vi "GE 5565PIORC.DMA.vi"(11 "count (1000)":i32=1000) -> (0 "error out":errorcluster, 3 "pass?":bool)   [LabVIEW 2016]
uses:
  <vilib>/NI/GE Reflective Memory Driver/GE 5565PIORC.lvclass/GE 5565PIORC.ctl
  <vilib>/NI/GE Reflective Memory Driver/Methods/GE 5565PIORC.DMA.Create Transfer (Block).vi
  <vilib>/NI/GE Reflective Memory Driver/Methods/GE 5565PIORC.DMA.Block.Read (DBL).vi
  <vilib>/NI/GE Reflective Memory Driver/Properties/Registers/GE 5565PIORC.Registers.INTCSR.Local DMA Channel 0 Interrupt Enable.Set.vi
  <vilib>/NI/GE Reflective Memory Driver/Properties/Registers/GE 5565PIORC.Registers.INTCSR.PCI Interrupt Enable.Set.vi
  <vilib>/NI/GE Reflective Memory Driver/Properties/Registers/GE 5565PIORC.Registers.INTCSR.Local Interrupt Input Enable.Set.vi
  <vilib>/NI/GE Reflective Memory Driver/Properties/Registers/GE 5565PIORC.Registers.DMACSR0.Channel 0 Enable.Set.vi
  <vilib>/NI/GE Reflective Memory Driver/Methods/GE 5565PIORC.DMA.Create Transfer (Scatter-Gather).vi
  <vilib>/NI/GE Reflective Memory Driver/Methods/GE 5565PIORC.PXI Interrupts.Discard Events.vi
  <vilib>/NI/GE Reflective Memory Driver/Methods/GE 5565PIORC.DMA.Start.vi
  <vilib>/NI/GE Reflective Memory Driver/Methods/GE 5565PIORC.DMA.Wait for Done Interrupt.vi
  <vilib>/NI/GE Reflective Memory Driver/Methods/GE 5565PIORC.VISA.Move In.DBL.vi
  <vilib>/NI/GE Reflective Memory Driver/Properties/Registers/GE 5565PIORC.Registers.Local Configuration.Read.vi
  <vilib>/NI/GE Reflective Memory Driver/Properties/Registers/GE 5565PIORC.Registers.Local Configuration.Read (U32).vi
  <vilib>/NI/GE Reflective Memory Driver/Properties/Registers/GE 5565PIORC.Registers.Local Configuration.Write.vi
  <vilib>/NI/GE Reflective Memory Driver/Properties/Registers/GE 5565PIORC.Registers.Local Configuration.Write (U32).vi
  <vilib>/NI/GE Reflective Memory Driver/Methods/GE 5565PIORC.Bit Manipulation.Set Bit.vi
  <vilib>/NI/GE Reflective Memory Driver/Methods/GE 5565PIORC.Bit Manipulation.Set Bit (U32).vi
  <vilib>/NI/GE Reflective Memory Driver/Properties/Registers/GE 5565PIORC.Registers.Local Configuration.Read (U8).vi
  <vilib>/NI/GE Reflective Memory Driver/Properties/Registers/GE 5565PIORC.Registers.Local Configuration.Write (U8).vi
  <vilib>/NI/GE Reflective Memory Driver/Methods/GE 5565PIORC.Bit Manipulation.Set Bit (U8).vi
  <vilib>/NI/GE Reflective Memory Driver/Methods/GE 5565PIORC.DMA.Size.vi
  <vilib>/Utility/error.llb/Clear Errors.vi
  <vilib>/NI/GE Reflective Memory Driver/Properties/Registers/GE 5565PIORC.Registers.DMACSR0.Channel 0 Start.Set.vi
  <vilib>/NI/GE Reflective Memory Driver/Methods/GE 5565PIORC.PXI Interrupts.Wait for Event.vi
  <vilib>/NI/GE Reflective Memory Driver/Properties/Registers/GE 5565PIORC.Registers.DMACSR0.Channel 0 Clear Interrupt.Set.vi
  <vilib>/NI/GE Reflective Memory Driver/Methods/GE 5565PIORC.VISA.Move In.String (U8).vi
  <vilib>/NI/GE Reflective Memory Driver/Methods/GE 5565PIORC.Registers.Read.vi
  <vilib>/NI/GE Reflective Memory Driver/Methods/GE 5565PIORC.Registers.Read (U32).vi
  <vilib>/NI/GE Reflective Memory Driver/Methods/GE 5565PIORC.Registers.Write.vi
  <vilib>/NI/GE Reflective Memory Driver/Methods/GE 5565PIORC.Registers.Write (U32).vi
  <vilib>/NI/GE Reflective Memory Driver/Methods/GE 5565PIORC.Registers.Read (U8).vi
  <vilib>/NI/GE Reflective Memory Driver/Methods/GE 5565PIORC.Registers.Write (U8).vi
  <vilib>/NI/GE Reflective Memory Driver/Methods/GE 5565PIORC.VISA.Return Handler.vi
  <vilib>/NI/GE Reflective Memory Driver/Methods/GE 5565PIORC.Round Up to Nearest 8.vi
  <vilib>/NI/GE Reflective Memory Driver/Methods/GE 5565PIORC.Round Up to Nearest 16.vi
  <vilib>/NI/GE Reflective Memory Driver/Methods/GE 5565PIORC.DMA.Block.Write (DBL).vi
  <vilib>/NI/GE Reflective Memory Driver/Methods/GE 5565PIORC.DMA.Configure.vi
  <vilib>/Utility/error.llb/Error Cluster From Error Code.vi
  <vilib>/NI/GE Reflective Memory Driver/GE 5565PIORC.lvclass
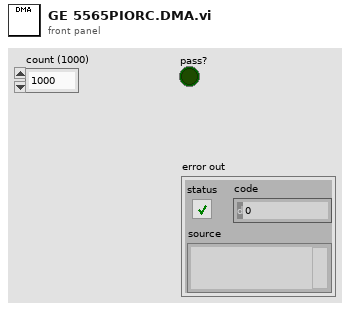
[diagram p1: front panel]
types:
  T1 = typedef "GE 5565PIORC.lvclass/GE 5565PIORC.Typedef.DMA Block Descriptor.ctl" = cluster{"descriptor ptr (VISA)":u32, "descriptor ptr (RFM)":u32, "descriptor size":u32, "descriptor params":T2}
  T2 = typedef "GE 5565PIORC.lvclass/GE 5565PIORC.Typedef.DMA Block Descriptor Params.ctl" = cluster{"data ptr (lower)":u32, "data ptr (upper)":u32, "data size":u32, "next descriptor ptr":u32}
  T3 = typedef "GE 5565PIORC.lvclass/GE 5565PIORC.Typedef.DMA Transfer Spec.ctl" = cluster{"RFM offset":u32, "Block Descriptors":T1[]}
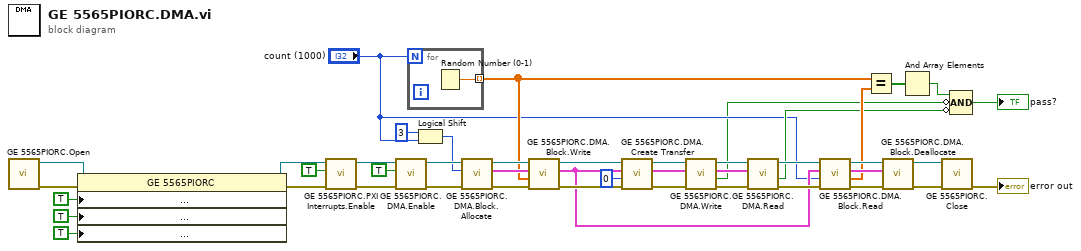
[diagram p0: block diagram]
diagram:
  n1 = call "GE 5565PIORC.Open.vi"() -> ("error out"=w11:errorcluster, "GE 5565PIORC"=w14:refnum<class "GE 5565PIORC.lvclass">)  [unwired: 10 in]
  n2 = property class="GE 5565PIORC"(reference=w14, error in=w11, "Properties:Board Registers:Local Configuration:03 - 0x68 - INTCSR:Local DMA Channel 0 Interrupt Enable"=TRUE ("Registers:Local Configuration:INTCSR:Local DMA Channel 0 Interrupt Enable"), "Properties:Board Registers:Local Configuration:03 - 0x68 - INTCSR:PCI Interrupt Enable"=TRUE ("Registers:Local Configuration:INTCSR:PCI Interrupt Enable"), "Properties:Board Registers:Local Configuration:03 - 0x68 - INTCSR:Local Interrupt Input Enable"=TRUE ("Registers:Local Configuration:INTCSR:Local Interrupt Input Enable")) -> (reference out=w13:refnum<class "GE 5565PIORC.lvclass">, error out=w12:errorcluster)
  n3 = call <vilib>:"GE 5565PIORC.PXI Interrupts.Enable.vi"("error in (no error)"=w12, "Enable Interrupts"=TRUE, "GE 5565PIORC in"=w13) -> ("error out"=w16:errorcluster, "GE 5565PIORC out"=w17:refnum<class "GE 5565PIORC.lvclass">)  [unwired: 7 in]
  n4 = call <vilib>:"GE 5565PIORC.DMA.Enable.vi"("error in (no error)"=w16, "Enable DMA"=TRUE, "GE 5565PIORC in"=w17) -> ("error out"=w41:errorcluster, "GE 5565PIORC out"=w42:refnum<class "GE 5565PIORC.lvclass">)  [unwired: 7 in]
  n5 = for {
    N: "count (1000)" -> [_]
    tunnel: [w45] -> w26 mode=indexing
    n6 = Random Number (0-1)() -> (number: 0 to 1=w45:dbl)
  }
  n7 = Logical Shift(y=i16 3, x="count (1000)") -> (x << y=w36:i32)
  n8 = call <vilib>:"GE 5565PIORC.DMA.Block.Allocate.vi"("error in (no error)"=w41, "size in bytes"=w36, "GE 5565PIORC in"=w42) -> ("error out"=w38:errorcluster, "Block Descriptor"=w37:T1, "GE 5565PIORC out"=w39:refnum<class "GE 5565PIORC.lvclass">)  [unwired: 6 in]
  n9 = call-poly <vilib>:"GE 5565PIORC.DMA.Block.Write.vi"("error in (no error)"=w38, "data"=w26, "Block Descriptor in"=w37, "GE 5565PIORC in"=w39) -> ("error out"=w33:errorcluster, "Block Descriptor out"=w30:T1, "GE 5565PIORC out"=w34:refnum<class "GE 5565PIORC.lvclass">)  [unwired: 4 in, 1 out]
  n10 = call-poly <vilib>:"GE 5565PIORC.DMA.Create Transfer.vi"("error in (no error)"=w33, "RFM offset"=u32 0, "Block Descriptor"=w30, "GE 5565PIORC in"=w34) -> ("error out"=w6:errorcluster, "DMA Transfer Spec"=w5:T3, "GE 5565PIORC out"=w7:refnum<class "GE 5565PIORC.lvclass">)  [unwired: 4 in, 1 out]
  n11 = call <vilib>:"GE 5565PIORC.DMA.Write.vi"("error in (no error)"=w6, "DMA Transfer Spec"=w5, "GE 5565PIORC in"=w7) -> ("error out"=w2:errorcluster, "timed out?"=w1:bool, "DMA Transfer Spec dup"=w4:T3, "GE 5565PIORC out"=w3:refnum<class "GE 5565PIORC.lvclass">)  [unwired: 5 in]
  n12 = call <vilib>:"GE 5565PIORC.DMA.Read.vi"("error in (no error)"=w2, "DMA Transfer Spec"=w4, "GE 5565PIORC in"=w3) -> ("error out"=w31:errorcluster, "timed out?"=w24:bool, "GE 5565PIORC out"=w32:refnum<class "GE 5565PIORC.lvclass">)  [unwired: 5 in, 1 out]
  n13 = call-poly <vilib>:"GE 5565PIORC.DMA.Block.Read.vi"("error in (no error)"=w31, "count"="count (1000)", "Block Descriptor in"=w30, "GE 5565PIORC in"=w32) -> ("error out"=w27:errorcluster, "data out"=w25:dbl[], "Block Descriptor out"=w28:T1, "GE 5565PIORC out"=w29:refnum<class "GE 5565PIORC.lvclass">)  [unwired: 4 in]
  n14 = Equal?(x=w26, y=w25) -> (x = y?=w23:bool[])
  n15 = call <vilib>:"GE 5565PIORC.DMA.Block.Deallocate.vi"("error in (no error)"=w27, "Block Descriptor"=w28, "GE 5565PIORC in"=w29) -> ("error out"=w20:errorcluster, "GE 5565PIORC out"=w21:refnum<class "GE 5565PIORC.lvclass">)  [unwired: 7 in]
  n16 = And Array Elements(Boolean array=w23) -> (logical AND=w22:bool)
  n17 = call "GE 5565PIORC.Close.vi"("error in (no error)"=w20, "GE 5565PIORC"=w21) -> ("error out"=→"error out":errorcluster)  [unwired: 9 in]
  n18 = Compound Arithmetic op=AND(w22, invert w1, invert w24) -> (→"pass?":bool)
